vi "Data Loop.vi"(11 "FPGA Ref":T1) -> (3 "FPGA Ref OUT":T1)   [LabVIEW 2013]
uses:
  Real-Time/Controls/RT FIFO Mode.ctl
  Controls/FPGA_Reference.ctl
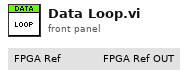
[diagram p1: front panel]
types:
  T1 = typedef "FPGA_Reference.ctl" = refnum<k20>
  T2 = typedef "RT FIFO Mode.ctl" = enum16{"Create", "Write", "Read", "Delete"}
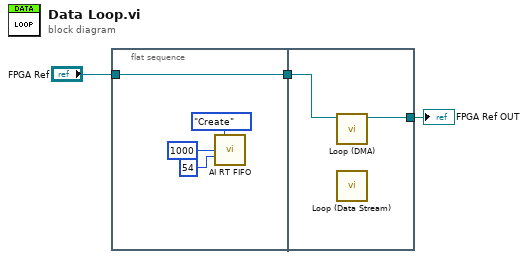
[diagram p0: block diagram]
diagram:
  n1 = flat-sequence {
    tunnel: [w7] -> w3
    tunnel: "FPGA Ref" -> [w7]
    tunnel: w3 -> [w9]
    tunnel: [w8] -> w1
    frame #0 {
      n2 = call "AI RT FIFO.vi"("Mode"=RT_FIFO_Mode."Create", "Buffer Size"=1000, "# of elements"=54) -> ()  [unwired: 10 in, 3 out]
    }
    frame #1 {
      n3 = call "Loop (DMA).vi"("FPGA Ref"=w9) -> ("FPGA Ref Out"=w8:T1)  [unwired: 9 in, 1 out]
      n4 = call "Loop (Data Stream).vi"() -> ()  [unwired: 11 in, 1 out]
    }
  }
  "FPGA Ref OUT" <- w1
